vi "Done_Programming.vi"(8 "error in (no error)":errorcluster, 10 "board_num":i32, 11 "path in":path) -> (0 "error out":errorcluster, 3 "path out":path)   [LabVIEW 2013, in "SpinAPI-20140801.lvlib"]
uses:
  SpinAPI-20140801.lvlib
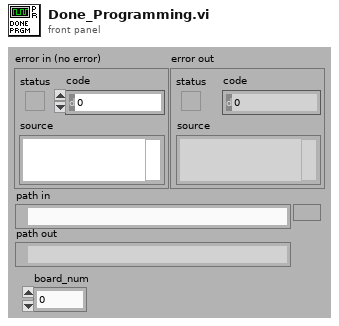
[diagram p1: front panel]
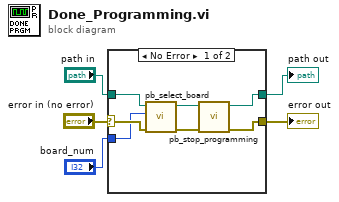
[diagram p0: block diagram]
diagram:
  n1 = case shown="No Error" "error in (no error)" {
    selector: "error in (no error)" -> [w12 w14]
    tunnel: [w7 w14] -> w4
    tunnel: "path in" -> [w11 w13]
    tunnel: [w6 w13] -> w2
    tunnel: "board_num" -> [w10 _]
    frame No Error {
      n2 = call "pb_select_board.vi"("error in (no error)"=w12, "board_num"=w10, "path in"=w11) -> ("error out"=w8:errorcluster, "path out"=w9:path)  [unwired: 7 in]
      n3 = call "pb_stop_programming.vi"("error in (no error)"=w8, "path in"=w9) -> ("error out"=w7:errorcluster, "path out"=w6:path)  [unwired: 8 in]
    }
    frame Error {
    }
  }
  "error out" <- w4
  "path out" <- w2
